vi "Flock_Shared_Delete Queue.vi"(8 "Error In":errorcluster, 11 "Process Name":T1) -> (0 "Error Out":errorcluster)   [LabVIEW 2014, in "Flock_Shared_Messaging.lvlib" / "Flock_Shared_LocalProcessMessaging.lvlib"]
uses:
  Flock_Shared_LocalProcessMessaging.lvlib
  Flock_Shared_Messaging.lvlib
  FGV_Action.ctl
  ProcessList.ctl
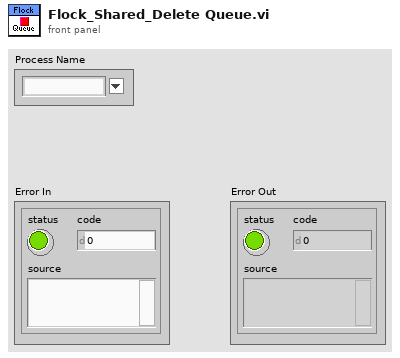
[diagram p1: front panel]
types:
  T1 = typedef "Flock_Shared_Messaging.lvlib/ProcessList.ctl" = string
  T2 = typedef "FGV_Action.ctl" = enum16{"Initalize Central", "Initialize Local", "Get", "Delete Local"}
  T3 = typedef "Flock_Shared_Messaging.lvlib/FGV_Queues.ctl" = cluster{"Local Queue in 2":T4, "Enum":T1}[]
  T4 = typedef "amc_Message Queue.ctl" = refnum<queue>
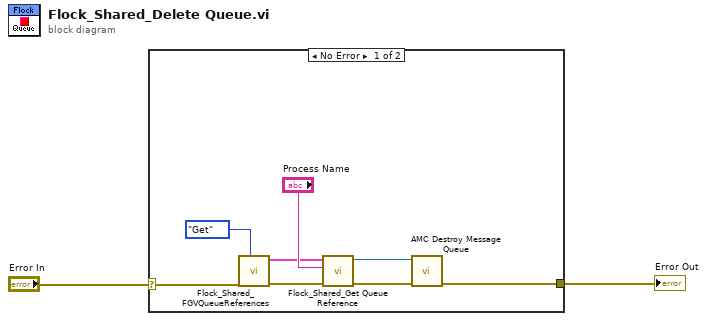
[diagram p0: block diagram]
diagram:
  n1 = case shown="No Error" "Error In" {
    selector: "Error In" -> [w9 w11]
    tunnel: [w8 w11] -> w1
    frame No Error {
      n2 = call "Flock_Shared_FGVQueueReferences.vi"("Action"=FGV_Action."Get", "error in (no error)"=w9) -> ("error out"=w6:errorcluster, "Array"=w4:T3)  [unwired: 7 in, 1 out]
      n3 = call "Flock_Shared_Get Queue Reference.vi"("Error In"=w6, "Enum"="Process Name", "Array"=w4) -> ("Error Out"=w7:errorcluster, "Local Queue out"=w3:T4)  [unwired: 7 in]
      n4 = call <vilib>:"AMC Destroy Message Queue.vi"("error in (no error)"=w7, "Message Queue in"=w3) -> ("error out"=w8:errorcluster)  [unwired: 8 in, 1 out]
    }
    frame Error {
    }
  }
  "Error Out" <- w1
